vi "exercicio_dropdown.vi"() -> ()   [LabVIEW 2020]
panel:
  in  "stop":bool
  out "Resultado":dbl
  in  "Entrada A":dbl
  in  "Entrada B":dbl
  in  "Operacao selecionada":T1(ring)
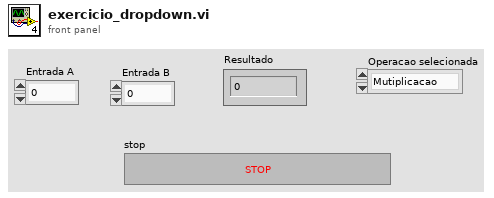
[diagram p1: front panel]
types:
  T1 = enum16{"Mutiplicacao", "subtracao", "DIvisão", "Soma"}
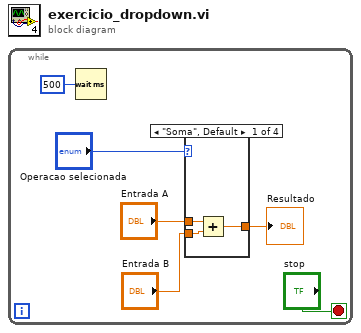
[diagram p0: block diagram]
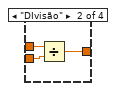
[diagram p2: hidden frame]
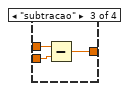
[diagram p3: hidden frame]
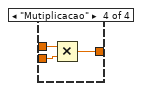
[diagram p4: hidden frame]
diagram:
  n1 = while {
    stop <- "stop" stop-if-true
    n2 = Wait (ms)(milliseconds to wait=u32 500) -> ()  [unwired: 1 out]
    n3 = case shown="\"Soma\", Default" "Operacao selecionada" {
      tunnel: [w9 w10 w15 w18] -> w5
      tunnel: "Entrada A" -> [w8 w12 w14 w17]
      tunnel: "Entrada B" -> [w7 w11 w13 w16]
      frame "Soma", Default {
        n4 = Add(x=w8, y=w7) -> (x+y=w9:dbl)
      }
      frame "DIvisão" {
        n5 = Divide(x=w12, y=w11) -> (x/y=w10:dbl)
      }
      frame "subtracao" {
        n6 = Subtract(x=w14, y=w13) -> (x-y=w15:dbl)
      }
      frame "Mutiplicacao" {
        n7 = Multiply(x=w17, y=w16) -> (x*y=w18:dbl)
      }
    }
    "Resultado" <- w5
  }
